vi "Insight_RW_Fixed_Wavelength_Power.vi"(7 "Parameter Type":enum16{"Value", "MAXimum", "MINimum", "DEFault"}(ring), 8 "error in (no error)":errorcluster, 9 "Mode (Read / Write)":enum8{"Write", "Read"}(ring), 10 "Power (mW)":dbl=1.0, 11 "telnet connection":T1) -> (0 "error out":errorcluster, 1 "response data":string, 2 "Power (mW) ?":dbl, 3 "telnet  connection out":T1)   [LabVIEW 2015]
doc: "Insight Photonic Solutions\n\nThis reads or write the power of the laser in Fixed Wavelength Mode. If you change the power, you need to run Power Calibration in Fixed Wavelength Mode to assure that all wavelengths are at the new power level.\n\nINPUTS:\nRead/Write : command or query the state of Fixed Wavelength Mode\nParameter Type - Tells the VI whether the command should use a Value or a keyword MAXimum, MINimum or DEFault to set the parameter value. (Default = Value).\nPower (mW): specify to within 1 uW precision (Default = 1mW)\n\nOUTPUTS:\nResponse Data - Entire string response from the laser\nPower (mW)? - power value in fixed wavelength mode, in mW, parsed from the total strung response\n\nver 1.0 - original release\nver 3.3 - changed parser to handle responses from Atlas ver 3.2 and earlier, and ver 3.3 and later\nver 3.4 - accepts key word values Max, Min or Default in addition to numeric values of the parameter"
uses:
  Telnet Session.ctl
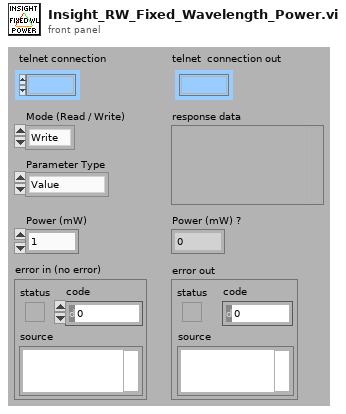
[diagram p1: front panel]
types:
  T1 = typedef "Telnet Session.ctl" = refnum<k1>
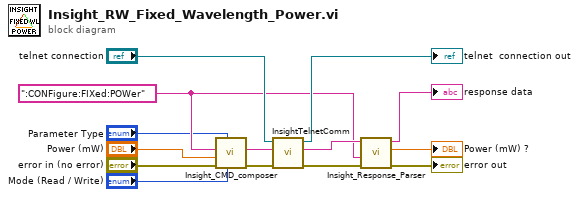
[diagram p0: block diagram]
diagram:
  w5 = ":CONFigure:FIXed:POWer" ("String")
  n1 = call "Insight_CMD_composer.vi"("Mode (Read / Write)"="Mode (Read / Write)", "Parameter Type"="Parameter Type", "error in (no error)"="error in (no error)", "Value"="Power (mW)", "CMD"=w5) -> ("error out"=w7:errorcluster, "Command String"=w6:string)  [unwired: 5 in]
  n2 = call "InsightTelnetComm.vi"("error in"=w7, "write buffer (\"\")"=w6, "telnet connection"="telnet connection") -> ("error out"=w12:errorcluster, "response data"=w8:string, "telnet  connection out"=→"telnet  connection out":T1)  [unwired: 4 in]
  n3 = call "Insight_Response_Parser.vi"("error in (no error)"=w12, "Command String"=w5, "Laser Response In"=w8) -> ("error out"=→"error out":errorcluster, "Value"=→"Power (mW) ?":dbl, "Laser Response Out"=→"response data":string)  [unwired: 6 in]
